vi "SetImageType.vi"(8 "error in (no error)":errorcluster, 10 "ImageType":T1, 11 "ICameraTestingProxy in":refnum<class "ICameraTestingProxy.lvclass">) -> (0 "error out":errorcluster, 3 "ICameraTestingProxy out":refnum<class "ICameraTestingProxy.lvclass">)   [LabVIEW 2020, in "ICameraTestingProxy.lvlib" / "ICameraTestingProxy.lvclass"]
uses:
  ICameraTestingProxy.lvclass
  TypeDef/ImageType.ctl
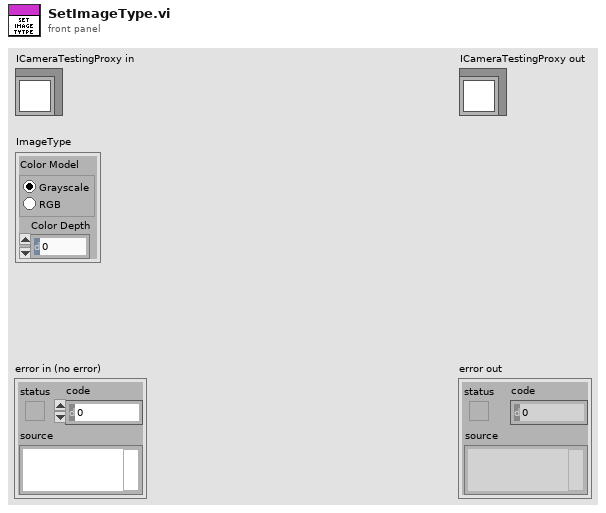
[diagram p1: front panel]
types:
  T1 = typedef "ICameraTestingProxy.lvlib/ICameraTestingProxy.lvclass/ImageType.ctl" = cluster{"Color Model":enum32{"GrayScale", "RGB"}, "Color Depth":u8}
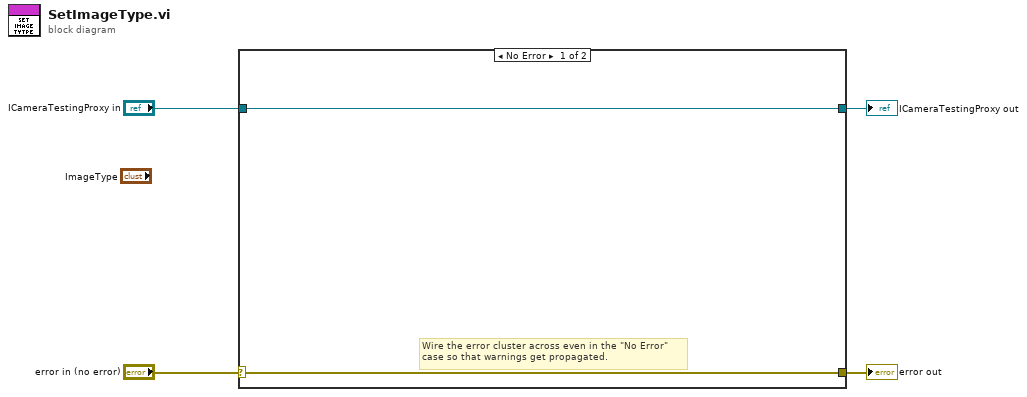
[diagram p0: block diagram]
diagram:
  n1 = case shown="No Error" "error in (no error)" {
    selector: "error in (no error)" -> [w5 w8]
    tunnel: [w5 w8] -> w3
    tunnel: [w6 w7] -> w1
    tunnel: "ICameraTestingProxy in" -> [w6 w7]
    frame No Error {
      # "Wire the error cluster across even in the \"No Error\"\ncase so that warnings get propagated."
    }
    frame Error {
    }
  }
  "error out" <- w3
  "ICameraTestingProxy out" <- w1
